vi "AlliGator Save Image Data to File.vi"(7 "Time Gate":u16, 8 "error in (no error)":errorcluster, 9 "Saved TIFF Image":T1=enum."Sum of All Gates" caption="Displayed Image", 10 "Image":T2, 11 "File Path in":path=path "") -> (0 "error out":errorcluster, 1 "Output String":string, 2 "Message":string, 3 "File Path out":path)   [LabVIEW 2021, in "AlliGator Files.lvlib"]
doc: "Saves <B>Original Image</B> to an image file using user-selected options."
uses:
  AlliGator Files.lvlib
  <vilib>/vision/Image Controls.llb/IMAQ Image.ctl
  AlliGator Saved TIFF Image Type.ctl
  Settings/AlliGator Settings List.ctl
  Settings/AlliGator Exported Image Settings.ctl
  <vilib>/Utility/error.llb/Error Cluster From Error Code.vi
  <vilib>/ErrorRing/Error Ring.xnode
  Settings/AlliGator Settings.lvlib
  Error/Error.lvlib
  Variant/Variant.lvlib
panel:
  # "see the AlliGator License on the block diagram (Ctrl+E or Window:Show Block Diagram)"
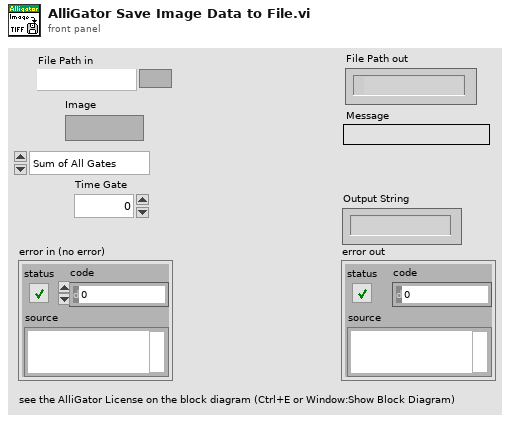
[diagram p1: front panel]
types:
  T1 = typedef "AlliGator Files.lvlib/AlliGator Saved TIFF Image Type.ctl" = enum16{"Single Gate", "Sum of All Gates", "Phasor"}
  T2 = typedef "IMAQ Image.ctl" = refnum<image>
  T3 = typedef "Phasor.lvlib/Phasor Fluorescence Lifetime Parameters v3.ctl" = cluster{"# Pixel X":i32, "# Pixel Y":i32, "# Gates":i32, "# Datasets":i32, "Gate Image Exposure":dbl[unit], "Macrotime Gate Separation":dbl[unit], "Nanotime Gate Separation":dbl[unit], "Gate Width":dbl[unit], "Laser Period":dbl[unit], "SYNC Period":dbl[unit], "Gate Image Integration":dbl[unit]}
  T4 = cluster{"Rows Per Strip":i32, "Photometric":i32, "Compression Type":i32}
  T5 = typedef "AlliGator Settings.lvlib/AlliGator Exported Image Settings.ctl" = cluster{"bitness":bool, " Min Value":sgl, " Max Value":sgl}
  T6 = typedef "AlliGator Settings.lvlib/AlliGator Settings List.ctl" = enum16{"GUI:Visible Settings Tab", "GUI:Last Run Version", "Source Image:Use Image Histogram for Contrast", "Source Image:Low Count Pixels Rejection Options", "Source Image:High Count Pixels Rejection Options", "Source Image:Use Image Brightness", "Source Image:Blend Overlay with Image Background", "Source Image:Use Fixed ROI Diameter", "Source Image:ROI Diameter", "Source Image:ROI Center Color", "Source Image:Peak Threshold", "Source Image:Intensity Threshold", "Source Image:Image Binning Options", "Source Image:Image Smoothing Options", "Source Image:Image Histogram Active", "Source Image:Invert Binary Mask", "Source Image:Hot Pixel Removal", "Source Image:Overlay Analyzed ROI Center", "Source Image:Auto-Adjust Contrast", "Source Image:Histogram Lower Percentile", "Source Image:Histogram Upper Percentile", "Source Image:Save Source Image", "Source Image:Scale Bar Options", "Source Image:Image Resolution (Pixel Size)", "Source Image:Flatfield Correction", "Source Image:Show Dead Left Columns Correction", "Source Image:Dead Left Columns Correction", "Source Image:Image Pre-Processing Operations Order", "Source Image:Overlay ROI Median", "Source Image:Median Overlay Color", "Data Information:Gate Width", "Data Information:Nanotime Gate Separation", "Data Information:Macrotime Gate Separation", "Data Information:Gate Step", "Data Information:# Gates", "Data Information:Gate Image Exposure", "Data Information:Gate Image Integration", "Data Information:Gates to Skip", "Data Information:Gates to Keep", "Data Information:Define Gates to", "Data Information:Channel Name", "Data Information:Available Channel Names", "Data Information:Channel Arithmetic", "Data Information:Background File Subtraction", "Data Information:Background File", "Data Information:Background Scaling Factor", "Data Information:Background Pile-up Correction", "Data Information:Background Pixel Well Capacity", "Data Information:Laser Period", "Data Information:SYNC Period", "Data Information:Pile-up Correction", "Data Information:Pixel Well Capacity", "Data Information:Dataset Scaling Factor", "Fluorescence Decay_Decay Pre-Processing:Reverse Gates", "Fluorescence Decay_Decay Pre-Processing:Verbose Decay Pre-Processing", "Fluorescence Decay_Decay Pre-Processing:Use Decay Pre-Processing", "Fluorescence Decay_Decay Pre-Processing:Background Subtraction", "Fluorescence Decay_Decay Pre-Processing:Background Definition Range", "Fluorescence Decay_Decay Pre-Processing:Baseline Subtraction Method", "Fluorescence Decay_Decay Pre-Processing:Decay Pre-Processing Operations Order", "Fluorescence Decay_Decay Pre-Processing:Smoothing Parameter", "Fluorescence Decay_Decay Pre-Processing:Shift Decay", "Fluorescence Decay_Decay Pre-Processing:Decay Shift Parameters", "Fluorescence Decay_Decay Pre-Processing:Fold Decay", "Fluorescence Decay_Decay Pre-Processing:# Folds", "Fluorescence Decay_Decay Pre-Processing:1-Normalize Decay", "Fluorescence Decay_Decay Pre-Processing:[0-1]-Normalize Decay", "Fluorescence Decay_Decay Pre-Processing:Smoothen Decay", "Fluorescence Decay_Decay Pre-Processing:Extrapolate Decay", "Fluorescence Decay_Decay Pre-Processing:Use Periodicity", "Fluorescence Decay_Decay Pre-Processing:Use Cursors", "Fluorescence Decay_Decay Pre-Processing:Tail Fraction", "Fluorescence Decay_Decay Pre-Processing:Head Fraction", "Fluorescence Decay_Decay Pre-Processing:Additional Points", "Fluorescence Decay_Decay Pre-Processing:Straighten Decay", "Fluorescence Decay_Decay Pre-Processing:Constant Background", "Fluorescence Decay_Decay Pre-Processing:Pixel-Normalize Decay", "Fluorescence Decay_Advanced Analysis:Extract IRF instead of Decay", "Fluorescence Decay_Advanced Analysis:IRF Extraction Options", "Fluorescence Decay_Advanced Analysis:IRF Optimization Options", "Fluorescence Decay_Advanced Analysis:Square Pulse Options", "Fluorescence Decay_Advanced Analysis:IRF Order", "Fluorescence Decay_Advanced Analysis:IRF Time Constants", "Fluorescence Decay_Advanced Analysis:Wavelet Analysis Options", "Fluorescence Decay_Advanced Analysis:Average Lifetime Options", "Fluorescence Decay_Fit Options:Fit Options", "Fluorescence Decay_Fit Options:Use Legacy Fitting Approach", "Fluorescence Decay_Fit Options:Use Data Information Laser Period", "Fluorescence Decay_Fit Parameters:Displayed Fit Parameters", "Fluorescence Decay_Fit Parameters:Fit Parameter Constraints", "Fluorescence Decay_Fit Parameters:Export Tabulated Results", "Fluorescence Decay_Fit Parameters:MLE Baseline Offset Type", "Fluorescence Decay_Fit Parameters:MLE Baseline Offset", "Fluorescence Decay_Fit Parameters:Guess Parameter Names", "Fluorescence Decay_Fit Parameters:Guess Parameter Values", "Fluorescence Decay_Fit Parameters:Guess Parameters Options", "Fluorescence Decay_Fit Parameters:Optimal Offset Selection Criterion", "Fluorescence Decay_Styles:Show Last Decay Only", "Fluorescence Decay_Styles:Decay Graph Color Array", "Fluorescence Decay:Decay Graph Active", "Fluorescence Decay Statistics:Min Peak Value", "Fluorescence Decay Statistics:Reject Low Decay Peak Pixels", "Fluorescence Decay Statistics:Reject High Decay Peak Pixels", "Fluorescence Decay Statistics:Max Peak Value", "Time Traces:Use File Timestamp", "Time Traces:Time Step", "Time Traces:Use Intensity Correction File", "Time Traces:Intensity Correction File", "Phasor Plot:Phasor Plot Smoothing Options", "Phasor Plot:Phasor Plot Size", "Phasor Plot:Phasor Plot Graphics Options", "Phasor Plot:Cumulative Phasor Plot", "Phasor Plot:Use Phasor Brightness", "Phasor Plot:Blend Overlay with Phasor Background", "Phasor Plot:Save Phasor Plot", "Phasor Plot:Show References", "Phasor Plot:Phasor Ratio Decay Range", "Phasor Plot:Exponential Fading", "Phasor Plot:Phasor Ratio Reference Colors", "Phasor Plot:Reference Radius", "Phasor Plot:Show Color Map Vertices", "Phasor Plot:Phasor Plot Active", "Phasor Plot:Phasor Ratio Color Map Type", "Phasor Plot:Phasor Ratio Color Map", "Phasor Plot:Phasor Ratio Display Range", "Phasor Plot:Selected Image ROI(s)", "Phasor Plot:All Image ROIs", "Phasor Plot:Selected Phasor Plot ROI(s)", "Phasor Plot:All Phasor Plot ROIs", "Phasor Plot:Phasor Ratio Color-Coded Quantity", "Phasor Plot:Store Phasor Harmonics", "Phasor Plot:Draw Reference Segment", "Phasor Plot:User-Defined Quantity", "Phasor Plot:Color Scale High Color", "Phasor Plot:Color Scale Low Color", "Phasor Graph:Phasor Frequency", "Phasor Graph:Phasor Ratio Type", "Phasor Graph:Pixel-level Phasor Computation", "Phasor Graph:Save Phasor Graph", "Phasor Graph:Phasor Graph Active", "Phasor Graph:Phasor SDV Options", "Phasor Calibration:Use Backup Calibration if needed", "Phasor Graph:Define Shortest Lifetime as", "Phasor Calibration:Backup Calibration Type", "Phasor Calibration:Calibration Type", "Phasor Calibration:Calibration Lifetime", "Phasor Calibration:Calibration Map Algorithm", "Single-Exponential Phasor Locus (SEPL):Gate Parameters", "Single-Exponential Phasor Locus (SEPL):User-defined Gate", "Single-Exponential Phasor Locus (SEPL):User-defined IRF", "Single-Exponential Phasor Locus (SEPL):Phasor Parameters", "Single-Exponential Phasor Locus (SEPL):Decay & IRF Parameters", "Single-Exponential Phasor Locus (SEPL):Display Parameters", "Lifetime Analysis:Decay Analysis Parameters", "Lifetime Analysis:Lifetime Map Active", "Plugins:Python Settings", "Miscellaneous:Verbose Mode", "Miscellaneous:Beep after Script", "Miscellaneous:Saved Image File Format", "Miscellaneous:Exported Gate Image Settings", "Miscellaneous:Include Loading in Timing", "Miscellaneous:Verbose Settings Mode", "Miscellaneous:Histogram Options", "Miscellaneous:Beep on Error", "Miscellaneous:# Logical Processors Used", "Miscellaneous:ROI Description Max Characters", "Miscellaneous:Verbose Error Mode", "Miscellaneous:Transparent Mask Color"}
  T7 = typedef "Image Type" = u32
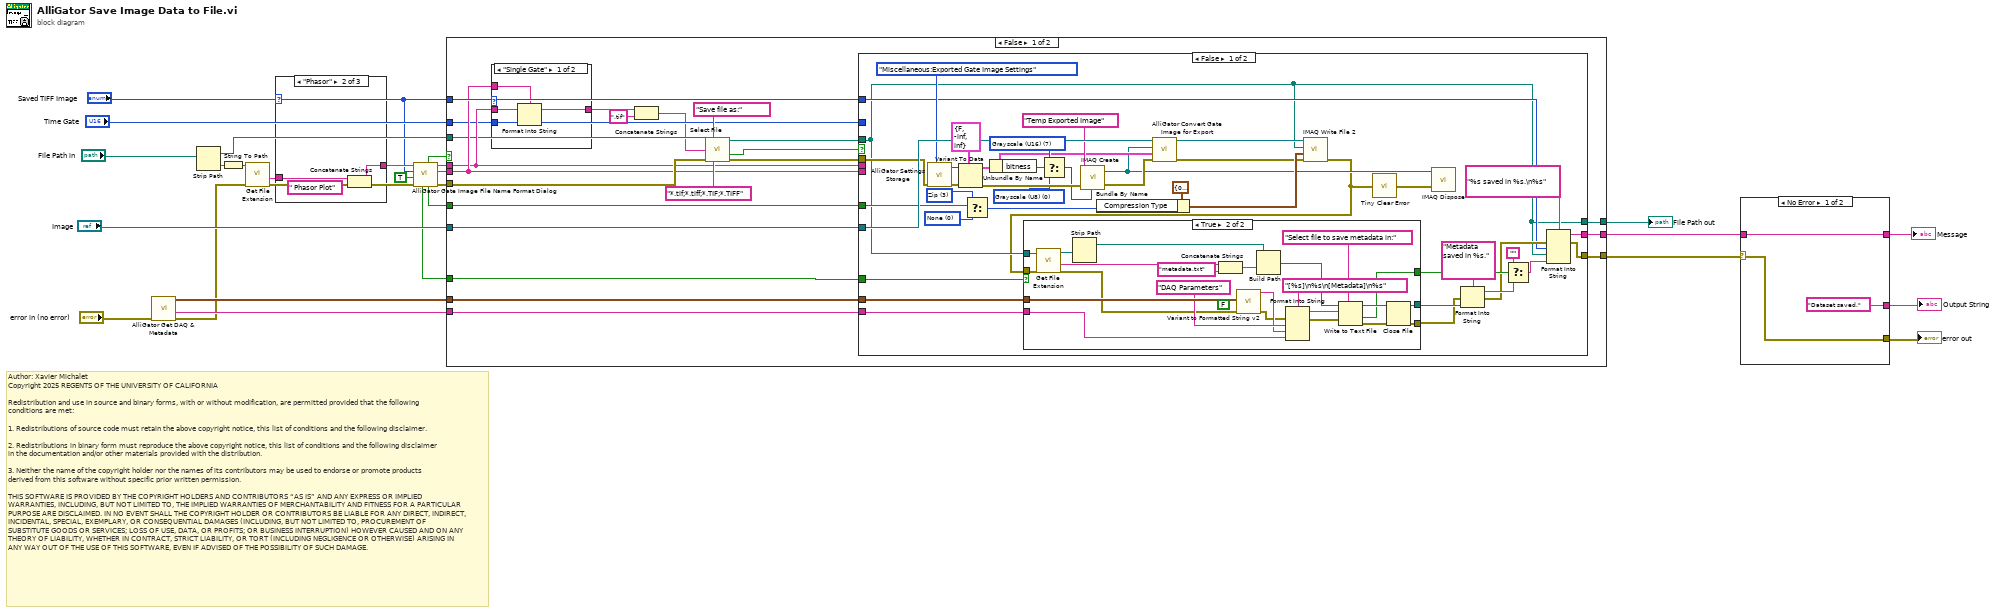
[diagram p0: block diagram]
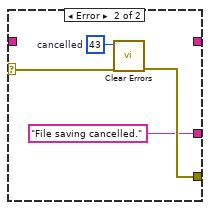
[diagram p2: hidden frame]
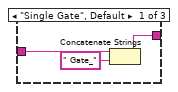
[diagram p3: hidden frame]
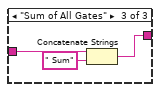
[diagram p4: hidden frame]
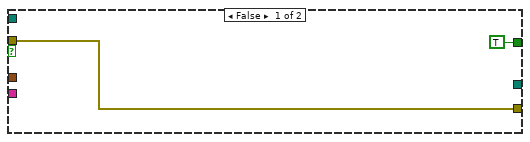
[diagram p6: hidden frame]
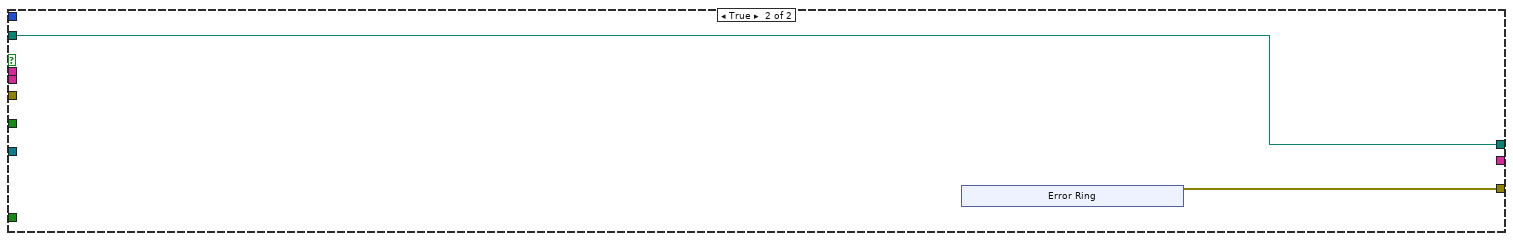
[diagram p8: hidden frame]
diagram:
  # "Author: Xavier Michalet\nCopyright 2025 REGENTS OF THE UNIVERSITY OF CALIFORNIA\n\nRedistribution and use in source and binary forms, with or without modification, are permitted provided that the following conditions are met:\n\n1. Redistributions of source code must retain the above copyright notice, this list of conditions and the following disclaimer.\n\n2. Redistributions in binary form must reproduce the above copyright notice, this list of conditions and the following disclaimer in the documentation and/or other materials provided with the distribution.\n\n3. Neither the name of the copyright holder nor the names of its contributors may be used to endorse or promote products derived from this software without specific prior written permission.\n\nTHIS SOFTWARE IS PROVIDED BY THE COPYRIGHT HOLDERS AND CONTRIBUTORS “AS IS” AND ANY EXPRESS OR IMPLIED WARRANTIES, INCLUDING, BUT NOT LIMITED TO, THE IMPLIED WARRANTIES OF MERCHANTABILITY AND FITNESS FOR A PARTICULAR PURPOSE ARE DISCLAIMED. IN NO EVENT SHALL THE COPYRIGHT HOLDER OR CONTRIBUTORS BE LIABLE FOR ANY DIRECT, INDIRECT, INCIDENTAL, SPECIAL, EXEMPLARY, OR CONSEQUENTIAL DAMAGES (INCLUDING, BUT NOT LIMITED TO, PROCUREMENT OF SUBSTITUTE GOODS OR SERVICES; LOSS OF USE, DATA, OR PROFITS; OR BUSINESS INTERRUPTION) HOWEVER CAUSED AND ON ANY THEORY OF LIABILITY, WHETHER IN CONTRACT, STRICT LIABILITY, OR TORT (INCLUDING NEGLIGENCE OR OTHERWISE) ARISING IN ANY WAY OUT OF THE USE OF THIS SOFTWARE, EVEN IF ADVISED OF THE POSSIBILITY OF SUCH DAMAGE."
  n1 = call "AlliGator Get DAQ & Metadata.vi"("Error In"="error in (no error)") -> ("Error Out"=w21:errorcluster, "Metadata"=w22:string, "DAQ Parameters"=w23:T3)  [unwired: 8 in]
  n2 = Strip Path(path="File Path in") -> (stripped path=w9:path, name=w17:string)
  n3 = String To Path(string=w17) -> (path=w15:path)
  n4 = call <vilib>:"Get File Extension.vi"("error in (no error)"=w21, "file"=w15) -> ("error out"=w16:errorcluster, "filename without extension"=w8:string)  [unwired: 5 in, 3 out]
  n5 = case shown="\"Phasor\"" "Saved TIFF Image" {
    tunnel: w8 -> [w29 w32 w36]
    tunnel: [w28 w31 w34] -> w7
    frame "Single Gate", Default {
      n6 = Concatenate Strings(w29, " Gate_" ("string")) -> (w28:string)
    }
    frame "Phasor" {
      n7 = Concatenate Strings(w32, " Phasor Plot" ("string")) -> (w31:string)
    }
    frame "Sum of All Gates" {
      n8 = Concatenate Strings(w36, " Sum" ("string")) -> (w34:string)
    }
  }
  n9 = call "AlliGator Gate Image File Name Format Dialog.vi"("error in (no error)"=w16, "Single Image"=TRUE, "Saved TIFF Image"="Saved TIFF Image", "Image File Name in"=w7) -> ("error out"=w18:errorcluster, "File Number Format out"=w19:string, "Gate Image File Name out"=w20:string, "Compress Image out"=w12:bool, "Cancelled?"=w14:bool, "Save Metadata File out"=w13:bool)  [unwired: 1 in, 1 out]
  n10 = case shown="False" w14 {
    tunnel: w20 -> [w42 _]
    tunnel: w19 -> [w43 _]
    tunnel: w18 -> [w58 _]
    tunnel: [w57 w133] -> w6
    tunnel: w9 -> [w38 w132]
    tunnel: [w55 w132] -> w26
    tunnel: [w56 _] -> w3
    tunnel: "Image" -> [w51 _]
    tunnel: w23 -> [w50 _]
    tunnel: w22 -> [w49 _]
    tunnel: w12 -> [w48 _]
    tunnel: w13 -> [w47 _]
    tunnel: "Time Gate" -> [w41 _]
    tunnel: "Saved TIFF Image" -> [w44 _]
    frame False {
      n11 = case shown="\"Single Gate\"" w44 {
        tunnel: w43 -> [w62 _]
        tunnel: w42 -> [w61 w63]
        tunnel: [w60 w63] -> w39
        tunnel: w41 -> [w59 _]
        frame "Single Gate" {
          n12 = Format Into String(format string=w62, initial string=w61, w59) -> (resulting string=w60:string)  [unwired: 1 in, 1 out]
        }
        frame "Sum of All Gates", Default {
        }
      }
      n13 = Concatenate Strings(w39, ".tif" ("string")) -> (w37:string)
      n14 = call "Select File"("start path"=w38, "prompt"="Save file as:", "default name"=w37, "error in"=w58, "pattern (all files)"="*.tif;*.tiff;*.TIF;*.TIFF") -> ("selected path"=w54:path, "cancelled"=w52:bool, "error out"=w53:errorcluster)  [unwired: 7 in, 1 out]
      n15 = case shown="False" w52 {
        tunnel: [w95 w130] -> w57
        tunnel: [w96 _] -> w56
        tunnel: [w66 w131] -> w55
        tunnel: w54 -> [w66 w131]
        tunnel: w53 -> [w74 w130]
        tunnel: w51 -> [w104 _]
        tunnel: w50 -> [w99 _]
        tunnel: w49 -> [w98 _]
        tunnel: w42 -> [_ _]
        tunnel: w43 -> [_ _]
        tunnel: w48 -> [w103 _]
        tunnel: w47 -> [w97 _]
        tunnel: w41 -> [_ _]
        tunnel: w44 -> [w69 _]
        frame False {
          w77 = T7 7 items=["Grayscale (U8)", "Grayscale (I16)", "Grayscale (SGL)", "Complex (CSG)", "RGB (U32)", "HSL (U32)", "RGB (U64)", "Grayscale (U16)"] ("Image Type")
          w78 = T7 0 items=["Grayscale (U8)", "Grayscale (I16)", "Grayscale (SGL)", "Complex (CSG)", "RGB (U32)", "HSL (U32)", "RGB (U64)", "Grayscale (U16)"] ("Image Type")
          w102 = 0 items=["None", "JPEG", "Run Length Encoded", "Zip"] ("Compression Type")
          w101 = 3 items=["None", "JPEG", "Run Length Encoded", "Zip"] ("Compression Type")
          n16 = call "AlliGator Settings Storage.vi"("AlliGator Settings List"=AlliGator_Settings_List."Miscellaneous:Exported Gate Image Settings", "Error In"=w74) -> ("Error Out"=w84:errorcluster, "Variant Data out"=w83:variant)  [unwired: 8 in]
          n17 = Variant To Data(error in=w84, type=T5 {"bitness"=FALSE, " Min Value"=-inf, " Max Value"=inf} ("Exported Gate Image Settings"), Variant=w83) -> (data=w73:T5, error out=w80:errorcluster)
          n18 = Select(t=w101, s=w103, f=w102) -> (s? t:f=w100:i32)
          n19 = Unbundle By Name(w73) -> ("bitness"=w81:bool)
          n20 = Select(t=w77, s=w81, f=w78) -> (s? t:f=w76:T7)
          n21 = call "IMAQ Create"("Image Name"="Temp Exported Image", "Image Type"=w76, "error in (no error)"=w80) -> ("New Image"=w67:T2, "error out"=w75:errorcluster)  [unwired: 2 in]
          n22 = Bundle By Name(cluster=T4 {"Rows Per Strip"=0, "Photometric"=1, "Compression Type"=0} ("TIFF Options"), "Compression Type"=w100) -> (w71:T4)
          n23 = call "AlliGator Convert Gate Image for Export.vi"("error in (no error)"=w75, "Exported Gate Image Settings"=w73, "Dest Image"=w67, "Original Image"=w104) -> ("error out"=w68:errorcluster, "Result Image"=w70:T2)  [unwired: 6 in]
          n24 = call-poly "IMAQ Write File 2"("error in (no error)"=w68, "TIFF Options"=w71, "File Path"=w66, "Image"=w70) -> ("error out"=w65:errorcluster)  [unwired: 6 in, 1 out]
          n25 = case shown="True" w97 {
            tunnel: w99 -> [_ w129]
            tunnel: w98 -> [_ w126]
            tunnel: w66 -> [_ w112]
            tunnel: [w105 w115] -> w91
            tunnel: [TRUE ("cancelled") w113] -> w90
            tunnel: [_ w114] -> w92
            tunnel: w65 -> [w105 w108]
            frame False {
            }
            frame True {
              (unwired) FALSE ("Hide Long Cluster Names (T)")
              n26 = call <vilib>:"Get File Extension.vi"("error in (no error)"=w108, "file"=w112) -> ("error out"=w107:errorcluster, "filename without extension"=w111:string, "dup file"=w110:path)  [unwired: 5 in, 2 out]
              n27 = Strip Path(path=w110) -> (stripped path=w109:path)  [unwired: 1 out]
              n28 = Concatenate Strings(w111, "metadata.txt" ("string")) -> (w120:string)
              n29 = call "Variant to Formatted String v2.vi"("error in (no error)"=w107, "Anything"=w129) -> ("error out"=w125:errorcluster, "String"=w127:string)  [unwired: 8 in]
              n30 = Build Path(base path=w109, name or relative path=w120) -> (appended path=w119:path)
              n31 = Format Into String(format string="[%s]\n%s\n[Metadata]\n%s", error in=w125, "DAQ Parameters" ("Label"), w127, w126) -> (resulting string=w123:string, error out=w122:errorcluster)  [unwired: 1 in]
              n32 = Write to Text File(prompt (Choose or enter file path)="Select file to save metadata in:", file (use dialog)=w119, text=w123, error in=w122) -> (refnum out=w117:refnum<file>, cancelled=w113:bool, error out=w116:errorcluster)
              n33 = Close File(refnum=w117, error in=w116) -> (path=w114:path, error out=w115:errorcluster)
            }
          }
          n34 = call "Tiny Clear Error.vi"("Error In"=w65) -> ("no Error Out"=w64:errorcluster)  [unwired: 8 in]
          n35 = call "IMAQ Dispose"("Image"=w67, "error in (no error)"=w64) -> ()  [unwired: 4 in, 1 out]
          n36 = Format Into String(format string="Metadata saved in %s.", error in=w91, w92) -> (resulting string=w89:string, error out=w88:errorcluster)  [unwired: 1 in]
          n37 = Select(t="", s=w90, f=w89) -> (s? t:f=w86:string)
          n38 = Format Into String(format string="%s saved in %s.\n%s", error in=w88, w69, w66, w86) -> (resulting string=w96:string, error out=w95:errorcluster)  [unwired: 1 in]
        }
        frame True {
        }
      }
    }
    frame True {
      n39 = xnode "Error Ring"() -> ("error out"=w133:errorcluster)
    }
  }
  "File Path out" <- w26
  n40 = case shown="No Error" w6 {
    selector: w6 -> [w138 w144]
    tunnel: [w138 w143] -> w4
    tunnel: ["Dataset saved." ("Output String") "File saving cancelled."] -> w5
    tunnel: w3 -> [w139 _]
    tunnel: [w139 _] -> w2
    frame No Error {
    }
    frame Error {
      w142 = 43  # cancelled
      n41 = call <vilib>:"Clear Errors.vi"("error in (no error)"=w144, "specific error code to clear (0: all)"=w142) -> ("error out"=w143:errorcluster)  [unwired: 4 in, 1 out]
    }
  }
  "error out" <- w4
  "Output String" <- w5
  "Message" <- w2
